vi "Untitled 1.07.vi"() -> ()   [LabVIEW 2019]
uses:
  <vilib>/rvi/Emulation/niFpgaGetClockAttributes.vi
  <vilib>/rvi/Emulation/niFpgaSctlEmulationGetInTimedLoop.vi
  <vilib>/rvi/Emulation/niFpgaEmulationReportErrorSimple.vi
  <vilib>/rvi/eio/common/nirviEmuTemplateMethod_errors.vi
  <vilib>/rvi/Emulation/niFpgaCriticalErrorInLSC.vi
  <vilib>/eio/EIONode/EIONode.xnode
panel:
  out "Count":i32
  out "Period":u32
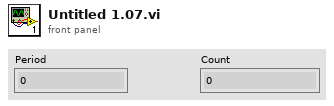
[diagram p1: front panel]
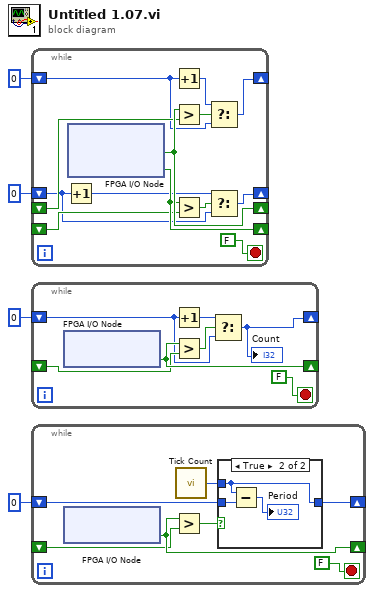
[diagram p0: block diagram]
diagram:
  n1 = while {
    shift-right: [w17] -> _
    shift-left: _ -> [w16]
    shift-right: [w15] -> _
    shift-left: _ -> [w14]
    shift-right: [w10] -> _
    shift-left: 0 ("x") -> [w11]
    shift-right: [w9] -> _
    shift-left: 0 ("x") -> [w8]
    stop <- FALSE stop-if-true
    n2 = Increment(x=w8) -> (x+1=w7:i32)
    n3 = xnode "FPGA I/O Node"() -> ("Mod8/DI0"=w17:bool, "Mod8/DI2"=w15:bool)  [unwired: 2 in, 2 out]
    n4 = Increment(x=w11) -> (x+1=w12:i32)
    n5 = Greater?(x=w17, y=w16) -> (0:w13:bool)
    n6 = Greater?(x=w15, y=w14) -> (0:w6:bool)
    n7 = Select(t=w12, s=w13, f=w11) -> (s? t:f=w10:i32)
    n8 = Select(t=w7, s=w6, f=w8) -> (s? t:f=w9:i32)
  }
  n9 = while {
    shift-right: [w24] -> _
    shift-left: _ -> [w23]
    shift-right: [w20] -> _
    shift-left: 0 ("x") -> [w21]
    stop <- FALSE stop-if-true
    n10 = xnode "FPGA I/O Node"() -> ("Mod8/DI1"=w24:bool)  [unwired: 1 in, 1 out]
    n11 = Increment(x=w21) -> (x+1=w22:i32)
    n12 = Greater?(x=w24, y=w23) -> (0:w18:bool)
    n13 = Select(t=w22, s=w18, f=w21) -> (s? t:f=w20:i32)
    "Count" <- w20
  }
  n14 = while {
    shift-right: [w31] -> _
    shift-left: _ -> [w30]
    shift-right: [w28] -> _
    shift-left: u32 0 ("Tick Count(mSec)") -> [w27]
    stop <- FALSE stop-if-true
    n15 = xnode "FPGA I/O Node"() -> ("Mod8/DI1"=w31:bool)  [unwired: 1 in, 1 out]
    n16 = Greater?(x=w31, y=w30) -> (0:w25:bool)
    n17 = call "Tick Count"() -> ("Tick Count(mSec)"=w26:u32)
    n18 = case shown="True" w25 {
      tunnel: w26 -> [_ w35]
      tunnel: [w32 w35] -> w28
      tunnel: w27 -> [w32 w34]
      frame False {
      }
      frame True {
        n19 = Subtract(x=w35, y=w34) -> (x-y=→"Period":u32)
      }
    }
  }
